vi "performStack.vi"() -> ()   [LabVIEW 2015]
panel:
  in  "no imgs":i32
  in  "inc.":dbl
  in  "axisIdx":i32
  in  "System no.":i32=1 min=1 max=4 step=1
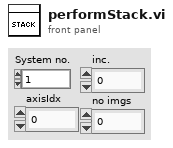
[diagram p1: front panel]
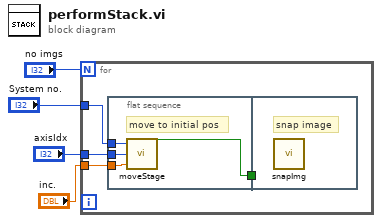
[diagram p0: block diagram]
diagram:
  n1 = for {
    N: "no imgs" -> [_]
    tunnel: "inc." -> [w8]
    tunnel: "axisIdx" -> [w7]
    tunnel: "System no." -> [w6]
    n2 = flat-sequence {
      tunnel: w8 -> [w12]
      tunnel: w7 -> [w11]
      tunnel: w6 -> [w10]
      tunnel: [w9] -> w5
      tunnel: w5 -> [_]
      frame #0 {
        # "move to initial pos"
        n3 = call "moveStage.vi"("inc (mm)"=w12, "axisIdx"=w11, "System no."=w10) -> ("Stopped"=w9:bool)
      }
      frame #1 {
        # "snap image"
        n4 = call "snapImg.vi"() -> ()  [unwired: 12 in]
      }
    }
  }
